vi "Pre-decoder.vi"(10 "Command window":string, 11 "offset in":i32) -> (0 "Command picked with code":string, 1 "code":string, 2 "Command picked":string, 3 "offset out":i32, 4 "remaining string":string)   [LabVIEW 2017]
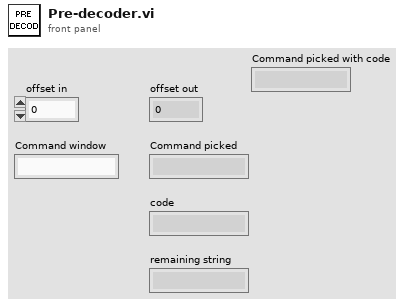
[diagram p1: front panel]
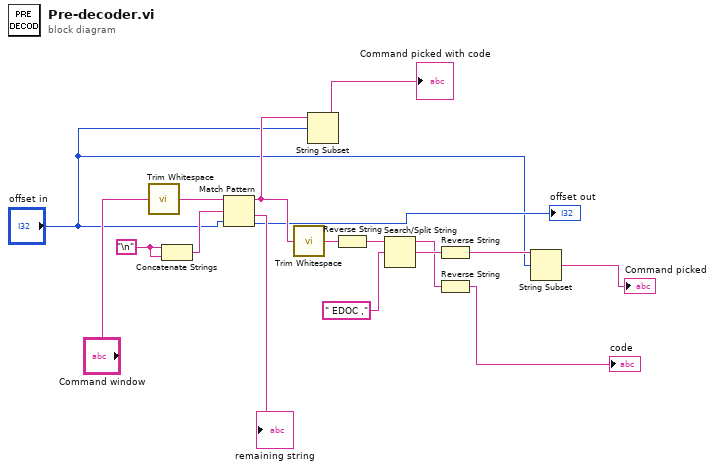
[diagram p0: block diagram]
diagram:
  w6 = "\n"
  n1 = call <vilib>:"Trim Whitespace.vi"("string"="Command window") -> ("trimmed string"=w16:string)  [unwired: 1 in]
  n2 = Concatenate Strings(w6, w6) -> (w5:string)
  n3 = Match Pattern(string=w16, regular expression=w5, offset (0)="offset in") -> (before substring=w8:string, after substring=→"remaining string":string, offset past match=→"offset out":i32)  [unwired: 1 out]
  n4 = call <vilib>:"Trim Whitespace.vi"("string"=w8) -> ("trimmed string"=w9:string)  [unwired: 1 in]
  n5 = String Subset(string=w8, offset (0)="offset in") -> (substring=→"Command picked with code":string)  [unwired: 1 in]
  n6 = Reverse String(1:w9) -> (0:w10:string)
  n7 = Search/Split String(string=w10, search string/char (-)=" EDOC ,") -> (substring before match=w12:string, match + rest of string=w13:string)  [unwired: 1 in, 1 out]
  n8 = Reverse String(1:w13) -> (0:w3:string)
  n9 = Reverse String(1:w12) -> (0:→"code":string)
  n10 = String Subset(string=w3, offset (0)="offset in") -> (substring=→"Command picked":string)  [unwired: 1 in]
